vi "checkQueue.vi"(8 "error in (no error)":errorcluster, 11 "ParameterConf in":refnum<class "ParameterConf.lvclass">) -> (0 "error out":errorcluster, 1 "Numeric":i16, 3 "ParameterConf out":refnum<class "ParameterConf.lvclass">)   [LabVIEW 2017, in "LibraryGcode.lvlib" / "ParameterConf.lvclass"]
uses:
  ParameterConf.lvclass
  ParameterConf.lvclass/ParameterConf.ctl
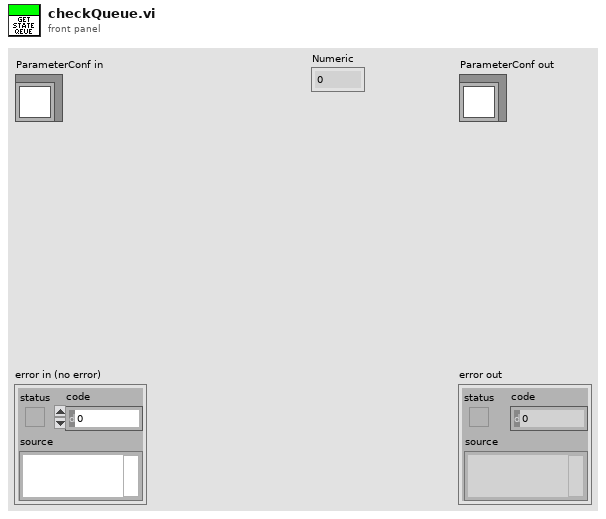
[diagram p1: front panel]
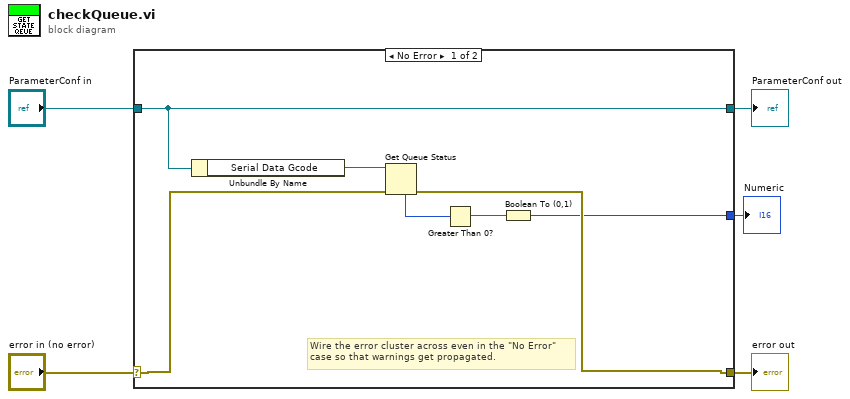
[diagram p0: block diagram]
diagram:
  n1 = case shown="No Error" "error in (no error)" {
    selector: "error in (no error)" -> [w10 w14]
    tunnel: [w9 w14] -> w4
    tunnel: [w12 w13] -> w2
    tunnel: "ParameterConf in" -> [w12 w13]
    tunnel: [w6 _] -> w1
    frame No Error {
      # "Wire the error cluster across even in the \"No Error\"\ncase so that warnings get propagated."
      n2 = Unbundle By Name(w12) -> ("Serial Data Gcode"=w11:refnum<queue>)
      n3 = Get Queue Status(queue=w11, error in (no error)=w10) -> (error out=w9:errorcluster, # elements in queue=w8:i32)  [unwired: 1 in, 6 out]
      n4 = Greater Than 0?(x=w8) -> (x > 0?=w7:bool)
      n5 = Boolean To (0,1)(Boolean=w7) -> (0, 1=w6:i16)
    }
    frame Error {
    }
  }
  "error out" <- w4
  "ParameterConf out" <- w2
  "Numeric" <- w1
